vi "Target - REF - Working.vi"() -> ()   [LabVIEW 2015]
doc: "This VI first configures the sample clock on the module and starts it. Then it acquires single point data from four channels. In order for the loop rate to be synchronized with the module's clock, the data is pipelined before it is written it to a DMA FIFO so it can be transfered to the host."
uses:
  <vilib>/LabVIEW Targets/FPGA/cRIO/shared/nicrio_ModuleControls/nicrio_cRIO-9234_DataRatesRing2.ctl
  <vilib>/rvi/Emulation/niFpgaGetClockAttributes.vi
  <vilib>/rvi/Emulation/niFpgaSctlEmulationGetInTimedLoop.vi
  <vilib>/rvi/Emulation/niFpgaEmulationReportErrorSimple.vi
  <vilib>/rvi/eio/common/nirviEmuTemplateMethod_errors.vi
  <vilib>/rvi/eio/common/nirviEmuTemplatePropertyGet_noerrors.vi
  <vilib>/rvi/Emulation/niFpgaCriticalErrorInLSC.vi
  <vilib>/rvi/eio/common/nirviEmuTemplatePropertySet_errors.vi
  <vilib>/rvi/interface/RandomDataEmulation/niFpgaRandomDataHandleErrors.vi
  <vilib>/eio/EIOMethodNode/EIOMethodNode.xnode
  <vilib>/eio/EIOPropertyNode/EIOPropertyNode.xnode
  <vilib>/eio/EIONode/EIONode.xnode
  <vilib>/rvi/DataTransferAndStorage/Container/XNode/niFpgaContainer.xnode
  <vilib>/rvi/interface/RandomDataEmulation/nirviRandomDataFpgaReadWriteTemplate.vi
  <vilib>/rvi/eio/common/nirviEmuTemplatePropertyGet_errors.vi
  <vilib>/rvi/eio/common/nirviEmuTemplatePropertySet_noerrors.vi
  GPS Timekeeper Files/FPGA Timekeeper.lvlib
panel:
  out "FPGA Timekeeper time (ns)":u64
  out "GPS status":T1(ring)
  out "FPGA Timekeeper locked":bool
  out "offset from time reference":i32
  out "antenna status":T2(ring)
  out "satellites available":u8
  out "UTC offset":i8
  out "UTC offset valid":bool
  in  "Data Rate":T3=1 items=["51.200 kS/s (NI 9234)"=1, "25.600 kS/s (NI 9234)"=2, "17.067 kS/s (NI 9234)"=3, "12.800 kS/s (NI 9234)"=4, "10.240 kS/s (NI 9234)"=5, "8.533 kS/s (NI 9234)"=6, "7.314 kS/s (NI 9234)"=7, "6.400 kS/s (NI 9234)"=8, "5.689 kS/s (NI 9234)"=9, "5.120 kS/s (NI 9234)"=10, "4.654 kS/s (NI 9234)"=11, "4.267 kS/s (NI 9234)"=12, "3.938 kS/s (NI 9234)"=13, "3.657 kS/s (NI 9234)"=14, "3.413 kS/s (NI 9234)"=15, "3.200 kS/s (NI 9234)"=16, "3.012 kS/s (NI 9234)"=17, "2.845 kS/s (NI 9234)"=18, "2.695 kS/s (NI 9234)"=19, "2.560 kS/s (NI 9234)"=20, "2.438 kS/s (NI 9234)"=21, "2.328 kS/s (NI 9234)"=22, "2.226 kS/s (NI 9234)"=23, "2.133 kS/s (NI 9234)"=24, "2.048 kS/s (NI 9234)"=25, "1.969 kS/s (NI 9234)"=26, "1.896 kS/s (NI 9234)"=27, "1.829 kS/s (NI 9234)"=28, "1.765 kS/s (NI 9234)"=29, "1.707 kS/s (NI 9234)"=30, "1.652 kS/s (NI 9234)"=31]
  out "Acq Loop Ticks":u32
  out "FPGA Error":errorcluster
  out "Module Underflow":bool
  out "DMA FIFO Full":bool
  in  "Stop":bool
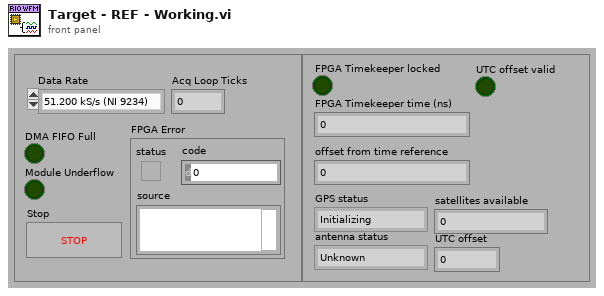
[diagram p1: front panel]
types:
  T1 = enum8{"Initializing", "Normal", "Unable to get fix"}
  T2 = enum8{"Unknown", "Normal", "Absent", "Overcurrent"}
  T3 = typedef "nicrio_cRIO-9234_DataRatesRing2.ctl" = u8
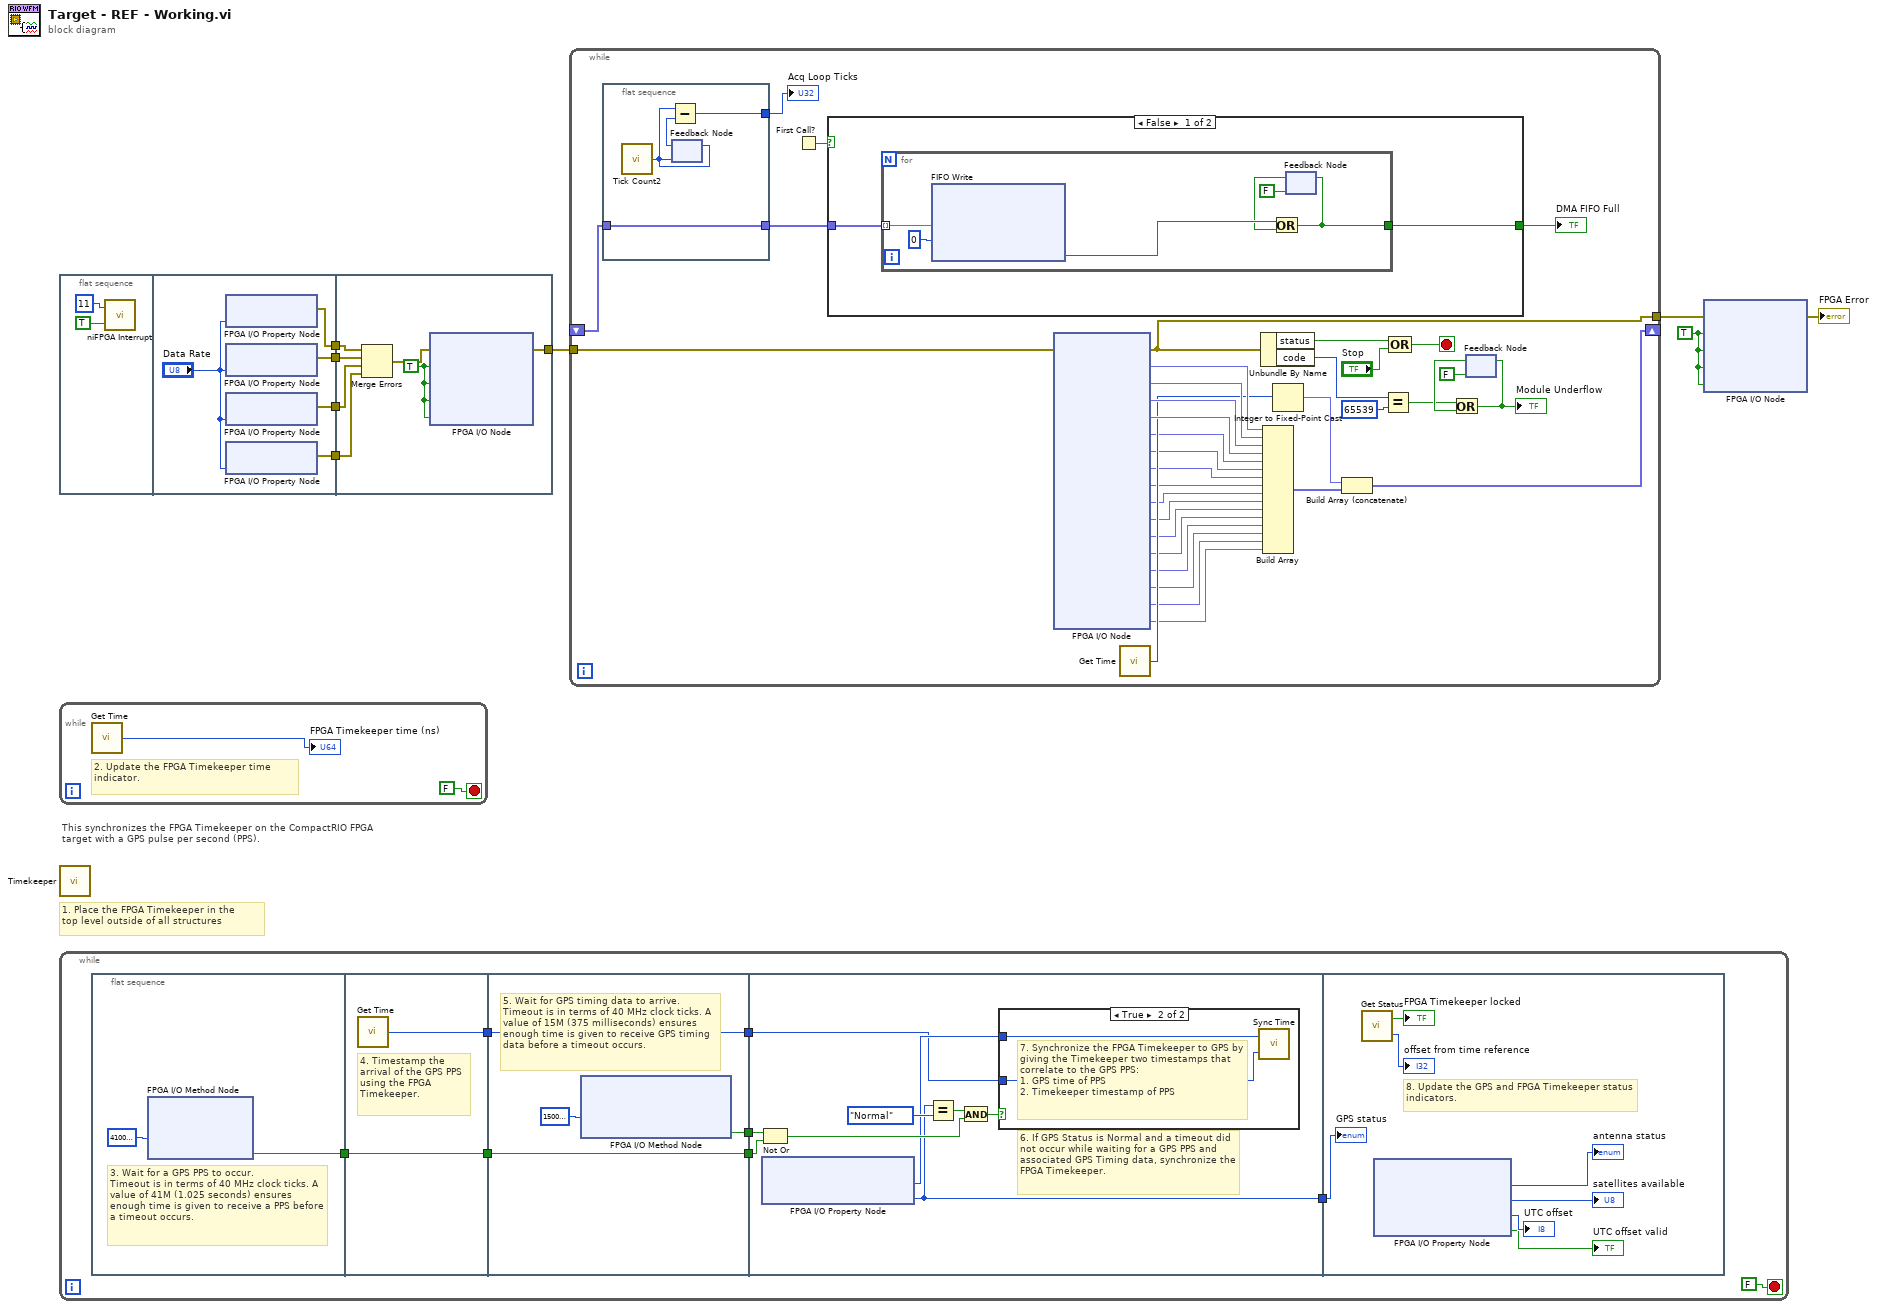
[diagram p0: block diagram]
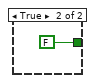
[diagram p3: hidden frame]
diagram:
  w1 = TRUE ("Mod1/Stop")
  # "This synchronizes the FPGA Timekeeper on the CompactRIO FPGA target with a GPS pulse per second (PPS)."
  # "1. Place the FPGA Timekeeper in the\ntop level outside of all structures"
  n1 = flat-sequence {
    tunnel: [w15] -> w5
    tunnel: [w13] -> w4
    tunnel: [w12] -> w3
    tunnel: [w11] -> w2
    tunnel: [w22] -> w8
    tunnel: w5 -> [w20]
    tunnel: w4 -> [w19]
    tunnel: w3 -> [w18]
    tunnel: w2 -> [w17]
    frame #0 {
      n2 = call <vilib>:"niFPGA Interrupt.vi"("Wait Until Cleared (F)"=TRUE ("Wait Until Cleared"), "IRQ Number (0)"=u8 11 ("IRQ Number")) -> ()  [unwired: 1 in]
    }
    frame #1 {
      n3 = xnode "FPGA I/O Property Node"("Data Rate"="Data Rate") -> ("error out"=w15:errorcluster)  [unwired: 2 in, 1 out]
      n4 = xnode "FPGA I/O Property Node"("Data Rate"="Data Rate") -> ("error out"=w13:errorcluster)  [unwired: 2 in, 1 out]
      n5 = xnode "FPGA I/O Property Node"("Data Rate"="Data Rate") -> ("error out"=w12:errorcluster)  [unwired: 2 in, 1 out]
      n6 = xnode "FPGA I/O Property Node"("Data Rate"="Data Rate") -> ("error out"=w11:errorcluster)  [unwired: 2 in, 1 out]
    }
    frame #2 {
      w16 = TRUE ("Mod1/Start")
      n7 = Merge Errors(w20, w19, w18, w17) -> (w21:errorcluster)
      n8 = xnode "FPGA I/O Node"("error in"=w21, "Mod4/Start"=w16, "Mod5/Start"=w16, "Mod6/Start"=w16, "Mod7/Start"=w16) -> ("error out"=w22:errorcluster)  [unwired: 4 in, 4 out]
    }
  }
  n9 = while {
    stop <- FALSE stop-if-true
    # "2. Update the FPGA Timekeeper time indicator."
    n10 = call "Get Time.vi"() -> ("time (ns)"=→"FPGA Timekeeper time (ns)":u64)  [unwired: 1 in]
  }
  n11 = call "Timekeeper.vi"() -> ()  [unwired: 12 in]
  n12 = while {
    stop <- FALSE stop-if-true
    n13 = flat-sequence {
      tunnel: [w33] -> w31
      tunnel: w31 -> [w36]
      tunnel: [w36] -> w30
      tunnel: [w35] -> w28
      tunnel: [w39] -> w32
      tunnel: w30 -> [w38]
      tunnel: [w38] -> w29
      tunnel: w28 -> [w37]
      tunnel: [w37] -> w27
      tunnel: w32 -> [w48]
      tunnel: w29 -> [w47]
      tunnel: w27 -> [w42]
      tunnel: [w41] -> w26
      tunnel: w26 -> [w58]
      frame #0 {
        # "3. Wait for a GPS PPS to occur.\nTimeout is in terms of 40 MHz clock ticks. A value of 41M (1.025 seconds) ensures enough time is given to receive a PPS before a timeout occurs."
        n14 = xnode "FPGA I/O Method Node"("Timeout"=41000000) -> ("Timed Out"=w33:bool)  [unwired: 1 in, 1 out]
      }
      frame #1 {
        # "4. Timestamp the arrival of the GPS PPS using the FPGA Timekeeper."
        n15 = call "Get Time.vi"() -> ("time (ns)"=w35:u64)  [unwired: 1 in]
      }
      frame #2 {
        # "5. Wait for GPS timing data to arrive.\nTimeout is in terms of 40 MHz clock ticks. A value of 15M (375 milliseconds) ensures enough time is given to receive GPS timing data before a timeout occurs."
        n16 = xnode "FPGA I/O Method Node"("Timeout"=15000000) -> ("Timed Out"=w39:bool)  [unwired: 1 in, 1 out]
      }
      frame #3 {
        # "6. If GPS Status is Normal and a timeout did not occur while waiting for a GPS PPS and associated GPS Timing data, synchronize the FPGA Timekeeper."
        n17 = Not Or(1:w47, 2:w48) -> (0:w45:bool)
        n18 = xnode "FPGA I/O Property Node"() -> ("PPS Timestamp (TAI)"=w43:u64, "GPS Status"=w41:T1)  [unwired: 1 in, 1 out]
        n19 = Equal?(x=w41, y=T1."Normal") -> (x = y?=w46:bool)
        n20 = And(x=w46, y=w45) -> (x .and. y?=w44:bool)
        n21 = case shown="True" w44 {
          tunnel: w43 -> [_ w51]
          tunnel: w42 -> [_ w50]
          frame False {
          }
          frame True {
            # "7. Synchronize the FPGA Timekeeper to GPS by giving the Timekeeper two timestamps that correlate to the GPS PPS:\n1. GPS time of PPS\n2. Timekeeper timestamp of PPS"
            n22 = call "Sync Time.vi"("FPGA Timekeeper time (ns)"=w50, "time reference time (ns)"=w51) -> ()
          }
        }
      }
      frame #4 {
        # "8. Update the GPS and FPGA Timekeeper status indicators."
        n23 = call "Get Status.vi"() -> ("FPGA Timekeeper locked"=→"FPGA Timekeeper locked":bool, "offset from time reference"=→"offset from time reference":i32)
        n24 = xnode "FPGA I/O Property Node"() -> ("Antenna Status"=→"antenna status":T2, "Satellites Available"=→"satellites available":u8, "UTC Offset"=→"UTC offset":i8, "UTC Offset Valid"=→"UTC offset valid":bool)  [unwired: 1 in, 1 out]
        "GPS status" <- w58
      }
    }
  }
  n25 = while {
    tunnel: [w90] -> w7
    shift-right: [w78] -> _
    shift-left: _ -> [w86]
    tunnel: w8 -> [w79]
    stop <- w93 stop-if-true
    n26 = flat-sequence {
      tunnel: [w105] -> w88
      tunnel: w86 -> [w104]
      tunnel: [w104] -> w87
      frame #0 {
        n27 = call "Tick Count2"() -> ("Tick Count(Ticks)"=w107:u32)
        n28 = feedback-in #1(w107) -> ()
        n29 = feedback #1(w107) -> (w106:u32)
        n30 = Subtract(x=w107, y=w106) -> (x-y=w105:u32)
      }
    }
    n31 = First Call?() -> (First Call?: T/F=w80:bool)
    n32 = case shown="False" w80 {
      tunnel: [w96 FALSE] -> w89
      tunnel: w87 -> [w95 _]
      frame False {
        n33 = for {
          tunnel: [w99] -> w96
          tunnel: w95 -> [w97] mode=indexing
          n34 = xnode ("FIFO Write")("Element"=w97, "Timeout"=0) -> ("Timed Out?"=w102:bool)  [unwired: 1 in, 1 out]
          n35 = feedback #2(FALSE) -> (w100:bool)
          n36 = Or(x=w102, y=w100) -> (x .or. y?=w99:bool)
          n37 = feedback-in #2(w99) -> ()
        }
      }
      frame True {
      }
    }
    "DMA FIFO Full" <- w89
    n38 = xnode "FPGA I/O Node"("error in"=w79) -> ("error out"=w90:errorcluster, "Mod4/AI0"=w75:fxp<+/-,24,4>, "Mod4/AI1"=w74:fxp<+/-,24,4>, "Mod4/AI2"=w73:fxp<+/-,24,4>, "Mod4/AI3"=w72:fxp<+/-,24,4>, "Mod5/AI0"=w70:fxp<+/-,24,4>, "Mod5/AI1"=w69:fxp<+/-,24,4>, "Mod5/AI2"=w68:fxp<+/-,24,4>, "Mod5/AI3"=w67:fxp<+/-,24,4>, "Mod6/AI0"=w66:fxp<+/-,24,4>, "Mod6/AI1"=w65:fxp<+/-,24,4>, "Mod6/AI2"=w64:fxp<+/-,24,4>, "Mod6/AI3"=w63:fxp<+/-,24,4>, "Mod7/AI0"=w62:fxp<+/-,24,4>, "Mod7/AI1"=w61:fxp<+/-,24,4>, "Mod7/AI2"=w60:fxp<+/-,24,4>, "Mod7/AI3"=w59:fxp<+/-,24,4>)  [unwired: 16 in, 16 out]
    n39 = call "Get Time.vi"() -> ("time (ns)"=w71:u64)  [unwired: 1 in]
    n40 = Unbundle By Name(w90) -> ("status"=w85:bool, "code"=w91:i32)
    n41 = Build Array(w75, w74, w73, w72, w70, w69, w68, w67, w66, w65, w64, w63, w62, w61, w60, w59) -> (w76:fxp<+/-,24,4>[])
    n42 = Integer to Fixed-Point Cast(integer=w71) -> (fixed-point=w77:fxp<+/-,64,44>)  [unwired: 1 in]
    n43 = Build Array (concatenate)(w77, w76) -> (w78:fxp<+/-,64,44>[])
    n44 = Equal?(x=w91, y=65539) -> (x = y?=w82:bool)
    n45 = Compound Arithmetic op=OR(w85, "Stop") -> (w93:bool)
    n46 = feedback #3(FALSE) -> (w84:bool)
    n47 = Or(x=w82, y=w84) -> (x .or. y?=w81:bool)
    "Module Underflow" <- w81
    n48 = feedback-in #3(w81) -> ()
    "Acq Loop Ticks" <- w88
  }
  n49 = xnode "FPGA I/O Node"("error in"=w7, "Mod4/Stop"=w1, "Mod5/Stop"=w1, "Mod6/Stop"=w1, "Mod7/Stop"=w1) -> ("error out"=→"FPGA Error":errorcluster)  [unwired: 4 in, 4 out]
